vi "ID_POS_SPEED_sync.vi"(8 "INVERSE":bool, 9 "speed":i32, 10 "Ax-Pos":i32, 11 "ID":u8) -> (3 "ID&POS&SPEED":u8[](array[numeric]) format="%x")   [LabVIEW 2017]
doc: "Output: [0]: ID\n [1]: POS_low_Byte\n [2]: POS_high_Byte\n [3]: Vel_low_Byte\n [4]: Vel_high_Byte"
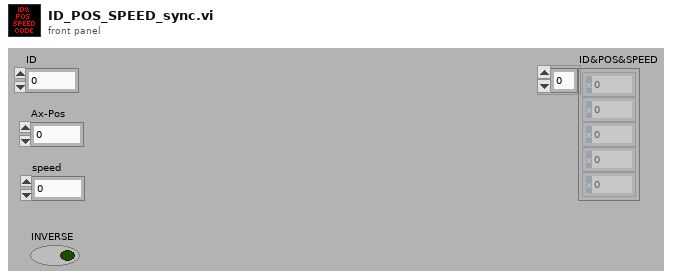
[diagram p1: front panel]
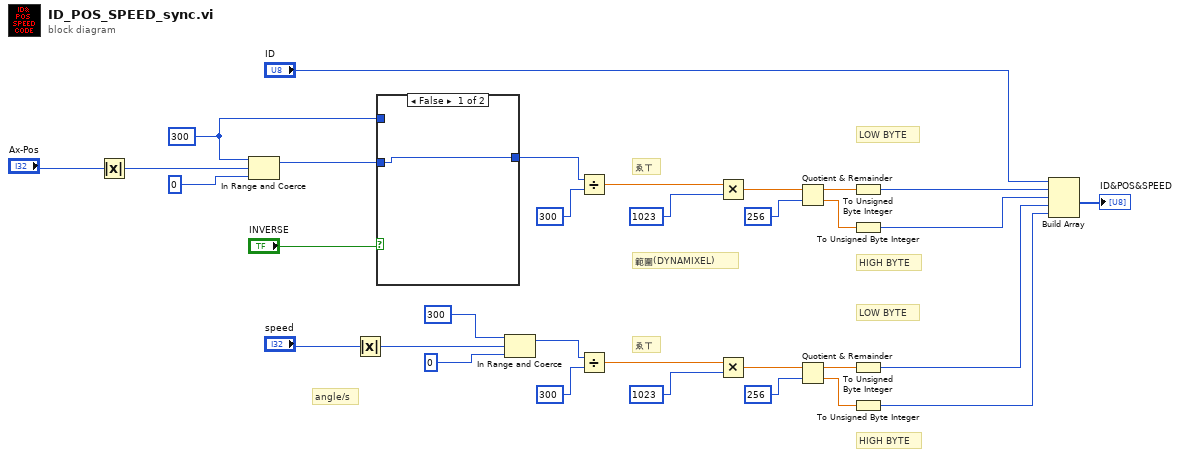
[diagram p0: block diagram]
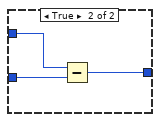
[diagram p2: hidden frame]
diagram:
  w2 = 300 ("upper limit")
  # "angle/s"
  # "ゑㄒ"
  # "HIGH BYTE"
  # "LOW BYTE"
  # "範圍(DYNAMIXEL)"
  # "ゑㄒ"
  # "HIGH BYTE"
  # "LOW BYTE"
  n1 = Absolute Value(x="Ax-Pos") -> (abs(x)=w31:i32)
  n2 = In Range and Coerce(upper limit=w2, x=w31, lower limit=0) -> (coerced(x)=w3:i32)  [unwired: 1 out]
  n3 = Absolute Value(x="speed") -> (abs(x)=w12:i32)
  n4 = case shown="False" "INVERSE" {
    tunnel: w3 -> [w33 w36]
    tunnel: w2 -> [_ w35]
    tunnel: [w33 w34] -> w1
    frame False {
    }
    frame True {
      n5 = Subtract(x=w35, y=w36) -> (x-y=w34:i32)
    }
  }
  n6 = In Range and Coerce(upper limit=300, x=w12, lower limit=0) -> (coerced(x)=w16:i32)  [unwired: 1 out]
  n7 = Divide(x=w1, y=300 ("upper limit")) -> (x/y=w28:dbl)
  n8 = Divide(x=w16, y=300 ("upper limit")) -> (x/y=w17:dbl)
  n9 = Multiply(x=w28, y=1023) -> (x*y=w26:dbl)
  n10 = Multiply(x=w17, y=1023) -> (x*y=w19:dbl)
  n11 = Quotient & Remainder(x=w26, y=256 ("upper limit")) -> (x-y*floor(x/y)=w23:dbl, floor(x/y)=w24:dbl)
  n12 = Quotient & Remainder(x=w19, y=256 ("upper limit")) -> (x-y*floor(x/y)=w22:dbl, floor(x/y)=w21:dbl)
  n13 = To Unsigned Byte Integer(number=w23) -> (unsigned 8bit integer=w10:u8)
  n14 = To Unsigned Byte Integer(number=w24) -> (unsigned 8bit integer=w9:u8)
  n15 = To Unsigned Byte Integer(number=w22) -> (unsigned 8bit integer=w8:u8)
  n16 = To Unsigned Byte Integer(number=w21) -> (unsigned 8bit integer=w7:u8)
  n17 = Build Array("ID", w10, w9, w8, w7) -> (→"ID&POS&SPEED":u8[])
